vi "update_weight_k.vi"(7 "t_k":dbl, 8 "O_k":dbl, 9 "Acc_input":dbl, 10 "eta":dbl) -> (1 "w_times_i":dbl, 3 "updated_weight":dbl)   [LabVIEW 2014]
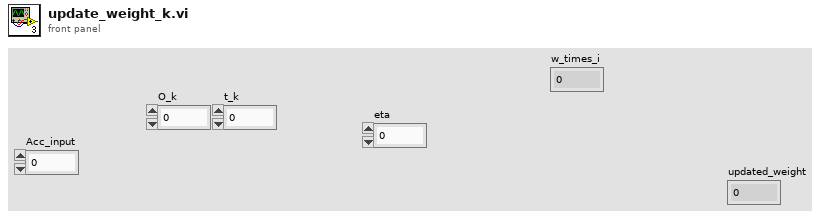
[diagram p1: front panel]
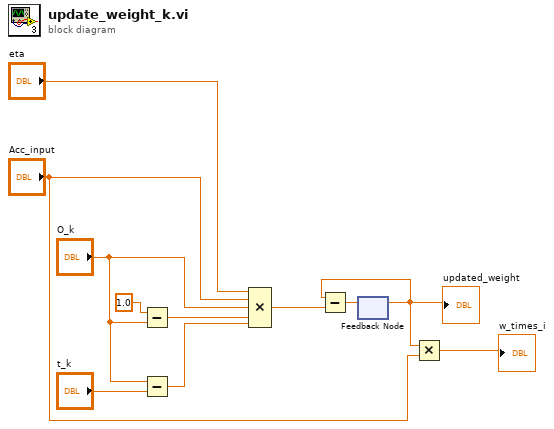
[diagram p0: block diagram]
diagram:
  n1 = Subtract(x=1.0, y="O_k") -> (x-y=w10:dbl)
  n2 = Subtract(x="O_k", y="t_k") -> (x-y=w8:dbl)
  n3 = Compound Arithmetic op=MULTIPLY("eta", "Acc_input", "O_k", w10, w8) -> (w7:dbl)
  n4 = feedback #1() -> (w2:dbl)  [unwired: 1 in]
  "updated_weight" <- w2
  n5 = Subtract(x=w2, y=w7) -> (x-y=w6:dbl)
  n6 = feedback-in #1(w6) -> ()
  n7 = Multiply(x=w2, y="Acc_input") -> (x*y=→"w_times_i":dbl)
